vi "ON-OFF Controller.vi"() -> ()   [LabVIEW 2014]
panel:
  in  "?":bool
  in  "Fan Control":bool
  in  "Heater Control":bool
  in  "Target":dbl(slide)=30.0 scale=0.0..60.0
  in  "Sample/ms":dbl(slide)=300.0 scale=0.0..20.0
  in  "Sensor Temperature":dbl(knob)=30.0 scale=0.0..60.0
  in  "?":bool
  out "Moderate":bool=TRUE
  out "Cold":bool
  out "Hot":bool
  out "Temperature Chart":dynamicdata(graph)
  in  "Minimum":dbl(slide)=25.26178010471204 scale=0.0..60.0
  in  "Maximum":dbl(slide)=35.026178010471206 scale=0.0..60.0
  out "Thermometer":dbl(slide)=30.0 scale=0.0..60.0
  # "ON/OFF Temperature Controller"
  # "Automatic"
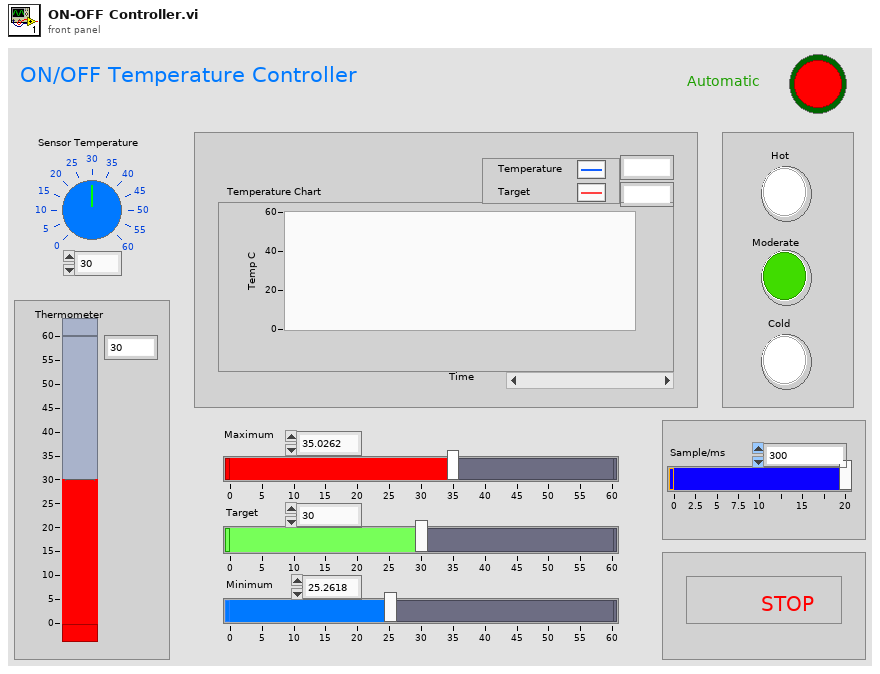
[diagram p1: front panel]
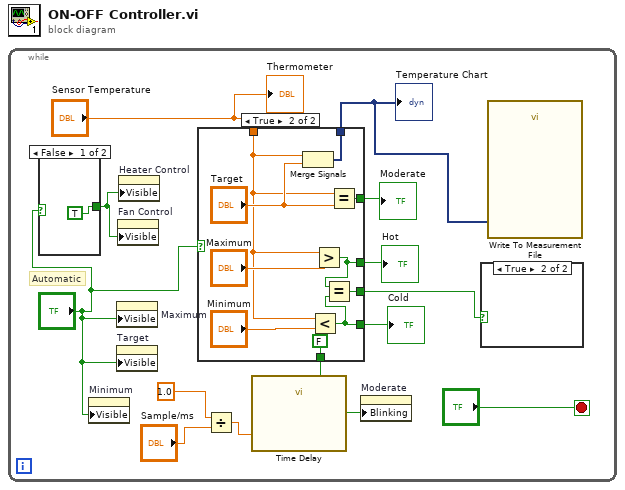
[diagram p0: block diagram]
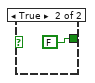
[diagram p2: hidden frame]
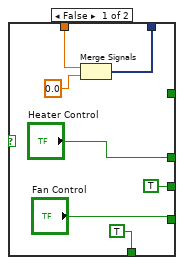
[diagram p3: hidden frame]
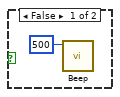
[diagram p4: hidden frame]
diagram:
  n1 = while {
    stop <- "?" stop-if-true
    # "Automatic"
    n2 = case shown="False" "?" {
      tunnel: [TRUE FALSE] -> w10
      frame False {
      }
      frame True {
      }
    }
    n3 = property on="Minimum" class="Slide (strict)"("Visible"="?") -> ()  [unwired: 2 in, 2 out]
    n4 = property on="Maximum" class="Slide (strict)"("Visible"="?") -> ()  [unwired: 2 in, 2 out]
    n5 = property on="Target" class="Slide (strict)"("Visible"="?") -> ()  [unwired: 2 in, 2 out]
    n6 = property on="Fan Control" class="Bool (strict)"("Visible"=w10) -> ()  [unwired: 2 in, 2 out]
    n7 = property on="Heater Control" class="Bool (strict)"("Visible"=w10) -> ()  [unwired: 2 in, 2 out]
    n8 = case shown="True" "?" {
      tunnel: "Sensor Temperature" -> [w22 w27]
      tunnel: [_ w30] -> w12
      tunnel: ["Heater Control" w25] -> w4
      tunnel: ["Fan Control" w24] -> w11
      tunnel: [w21 w28] -> w7
      tunnel: [TRUE FALSE] -> w6
      tunnel: [TRUE w23] -> w5
      frame False {
        n9 = Merge Signals(w22, 0.0) -> (w21:dynamicdata)
      }
      frame True {
        n10 = Merge Signals(w27, "Target") -> (w28:dynamicdata)
        n11 = Less?(x=w27, y="Minimum") -> (x < y?=w24:bool)
        n12 = Greater?(x=w27, y="Maximum") -> (0:w25:bool)
        n13 = Equal?(x=w25, y=w24) -> (x = y?=w23:bool)
        n14 = Equal?(x=w27, y="Target") -> (x = y?=w30:bool)
      }
    }
    "Hot" <- w4
    "Cold" <- w11
    "Temperature Chart" <- w7
    "Moderate" <- w12
    n15 = Divide(x=1.0, y="Sample/ms") -> (x/y=w1:dbl)
    n16 = call "Time Delay"("Delay Time (s)"=w1) -> ()  [unwired: 10 in, 1 out]
    n17 = property on="Moderate" class="Bool (strict)"("Blinking"=w6) -> ()  [unwired: 2 in, 2 out]
    n18 = case shown="True" w5 {
      frame False {
        n19 = call <vilib>:"Beep.vi"("frequency (Hz)"=u32 500) -> ()  [unwired: 11 in]
      }
      frame True {
      }
    }
    n20 = call "Write To Measurement File"("Signals"=w7) -> ()  [unwired: 16 in, 3 out]
    "Thermometer" <- "Sensor Temperature"
  }
